vi "Pcre2PatternOvectorInfo8.vi"(8 "error in":errorcluster, 11 "pCode":u64 format="%.0x") -> (0 "error out":errorcluster, 1 "OvectorSize":u64, 2 "OvectorEntries":u32, 3 "pCode":u64 format="%.0x", 5 "SubstringCount":u32)   [LabVIEW 2021, in "libpcre2-8.lvlib"]
uses:
  libpcre2-8.lvlib
  Pcre2FnkCallError.vi
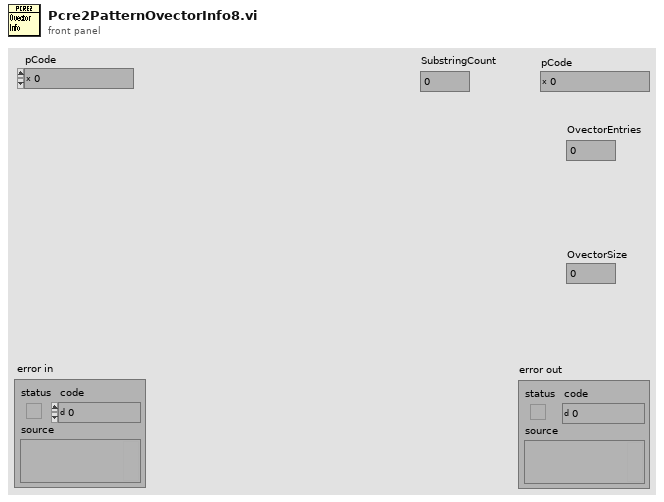
[diagram p1: front panel]
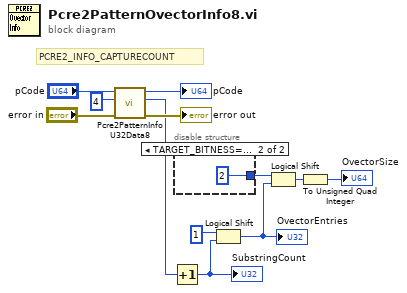
[diagram p0: block diagram]
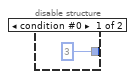
[diagram p2: hidden frame]
diagram:
  # "PCRE2_INFO_CAPTURECOUNT"
  n1 = call "Pcre2PatternInfoU32Data8.vi"("error in"="error in", "What"=u32 4, "pCode"="pCode") -> ("error out"=→"error out":errorcluster, "Info"=w1:u32, "pCode"=→"pCode":u64)  [unwired: 6 in]
  n2 = Increment(x=w1) -> (x+1=w9:u32)
  "SubstringCount" <- w9
  n3 = disable-structure shown="TARGET_BITNESS==32" {
    disable-tunnel: [i16 3 ("y") i16 2 ("y")] -> w12
    frame condition #0 {
    }
    frame condition #1 (active) {
    }
  }
  n4 = Logical Shift(y=i16 1, x=w9) -> (x << y=w10:u32)
  "OvectorEntries" <- w10
  n5 = Logical Shift(y=w12, x=w10) -> (x << y=w11:u32)
  n6 = To Unsigned Quad Integer(1:w11) -> (0:→"OvectorSize":u64)
